vi "PathPlanner_CommandUtil_DoNamed.vi"(11 "Event Action Name":string) -> ()   [LabVIEW 2019, in "PathPlanner24.lvlib"]
uses:
  PathPlanner24.lvlib
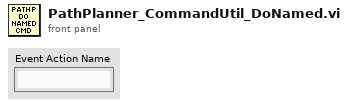
[diagram p1: front panel]
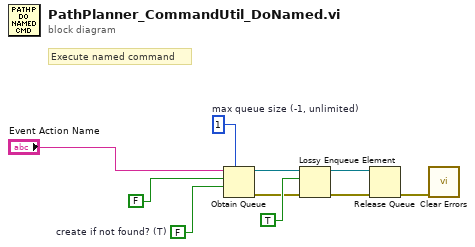
[diagram p0: block diagram]
diagram:
  w5 = FALSE  # create if not found? (T)
  w6 = 1  # max queue size (-1, unlimited)
  # "Execute named command"
  n1 = Obtain Queue(max queue size (-1, unlimited)=w6, name (unnamed)="Event Action Name", element data type=FALSE, create if not found? (T)=w5) -> (queue out=w2:refnum<queue>, error out=w1:errorcluster)  [unwired: 1 in, 1 out]
  n2 = Lossy Enqueue Element(queue=w2, element=TRUE, error in (no error)=w1) -> (queue out=w10:refnum<queue>, error out=w9:errorcluster)  [unwired: 2 out]
  n3 = Release Queue(queue=w10, error in (no error)=w9) -> (error out=w8:errorcluster)  [unwired: 1 in, 2 out]
  n4 = call <vilib>:"Clear Errors.vi"("error in (no error)"=w8) -> ()  [unwired: 5 in, 2 out]
